vi "Read Configuration Dictionary.vi"(8 "error in (no error)":errorcluster, 11 "ITestSettings in":refnum<class "ITestSettings.lvclass">) -> (0 "error out":errorcluster, 2 "Configuration Dictionary":variant, 3 "ITestSettings out":refnum<class "ITestSettings.lvclass">)   [LabVIEW 2016, in "ITestSettings.lvlib" / "ITestSettings.lvclass"]
uses:
  ITestSettings.lvclass
  ITestSettings.lvclass/ITestSettings.ctl
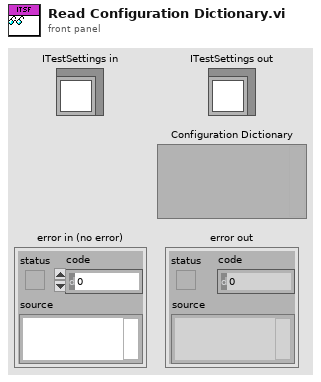
[diagram p1: front panel]
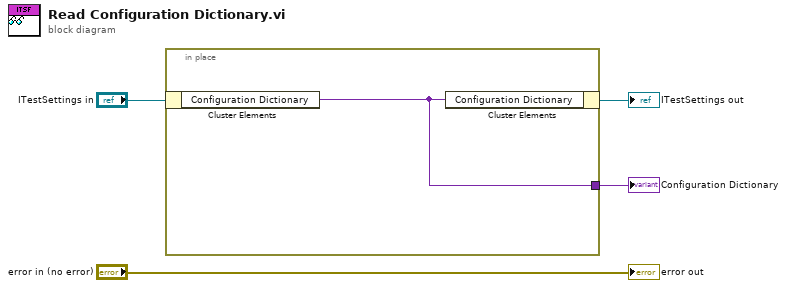
[diagram p0: block diagram]
diagram:
  n1 = in-place {
    in-place-border: [w5] -> w1
    n2 = in-place-cluster #1("ITestSettings in") -> ("Configuration Dictionary"=w5:variant)
    n3 = in-place-cluster #1("Configuration Dictionary"=w5) -> (→"ITestSettings out":refnum<class "ITestSettings.lvclass">)
  }
  "Configuration Dictionary" <- w1
  "error out" <- "error in (no error)"
